vi "GetStatus.vi"(8 "error in (no error)":errorcluster, 11 "AODAcq in":refnum<class "AODAcq.lvclass">) -> (0 "error out":errorcluster, 2 "Status":T2, 3 "AODAcq out":refnum<class "AODAcq.lvclass">)   [LabVIEW 2011, in "AODAcq.lvclass"]
uses:
  AODAcq.lvclass
  FPGA_Control/FPGAState.ctl
  <vilib>/rvi/interface/RandomDataEmulation/niFpgaReadControlTemplate.vi
  <vilib>/rvi/interface/nirviReadWriteControl/nirviReadWriteControl.xnode
  FPGA_Control/AODRef.ctl
  FPGA_Control/AOD Control (FPGA).vi
panel:
  out "Status.TemporalChFull":bool
  out "Scan.NumPoints":u32
  out "Status.DownsampleDone":bool
  out "Status.MotionChFull":bool
  out "Status.ImChFull":bool
  out "Scan.NumMotionPoints":u32
  out "Scan.Motion Increment":u32
  out "Scan.TotalSamples":u32
  out "Debug.PMT_Unpacked_backlog":u32
  out "Debug.PMT_Data_backlog":u32
  out "AOD.UpdatesPerPoint":u32=2000
  out "Comm.CommLines":enum16{"1", "2", "4"}(ring)
  out "Comm.WriteCount":i32
  out "Comm.Written":cluster{"Address":u8, "Value":u32}[](array[cluster])
  out "Debug.Point":cluster{"X":i32, "Y":i32, "Z":i32}
  out "Status.BufferedPoints":i32
  out "Debug.PMT_Samples":u32
  out "Scan.Samples":u32
  out "Debug.PMT Array":i32[](array[numeric])
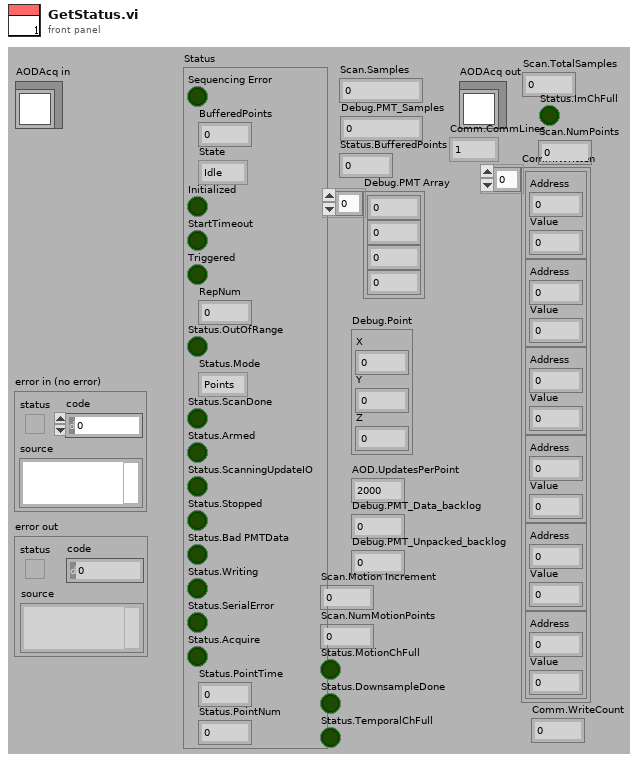
[diagram p1: front panel]
types:
  T1 = typedef "FPGAState.ctl" = enum16{"Idle", "Arm Scan", "Scan", "End Scan"}
  T2 = cluster{"Sequencing Error":bool, "BufferedPoints":i32, "State":T1, "Initialized":bool, "StartTimeout":bool, "Triggered":bool, "RepNum":u32, "Status.OutOfRange":bool, "Status.Mode":enum16{"Points", "Volume", "Idle"}, "Status.ScanDone":bool, "Status.Armed":bool, "Status.ScanningUpdateIO":bool, "Status.Stopped":bool, "Status.Bad PMTData":bool, "Status.Writing":bool, "Status.SerialError":bool, "Status.Acquire":bool, "Status.PointTime":u32, "Status.PointNum":u64}
  T3 = typedef "AODRef.ctl" = refnum<k20>
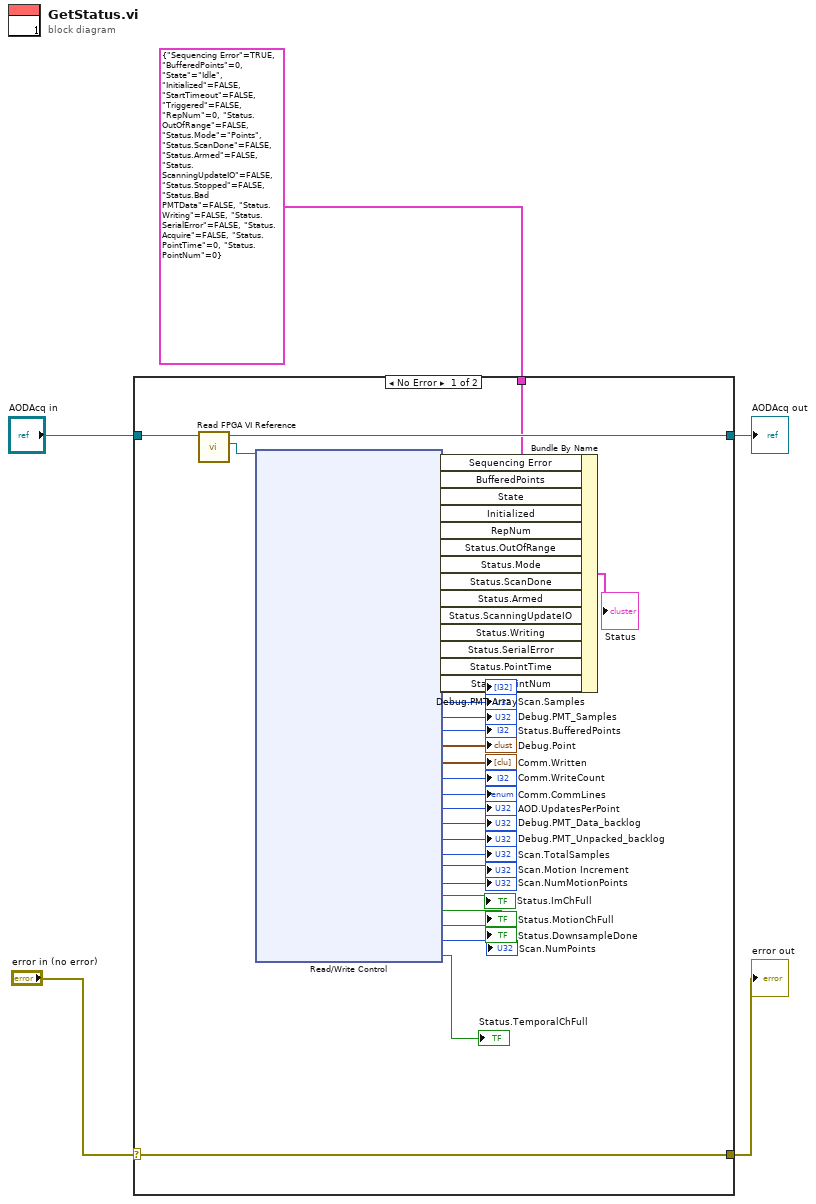
[diagram p0: block diagram]
diagram:
  n1 = case shown="No Error" "error in (no error)" {
    selector: "error in (no error)" -> [w44 w46]
    tunnel: [w44 w46] -> w4
    tunnel: [w42 w45] -> w2
    tunnel: "AODAcq in" -> [w43 w45]
    tunnel: T2 {"Sequencing Error"=TRUE, "BufferedPoints"=0, "State"=enum."Idle", "Initialized"=FALSE, "StartTimeout"=FALSE, "Triggered"=FALSE, "RepNum"=0, "Status.OutOfRange"=FALSE, "Status.Mode"=enum."Points", "Status.ScanDone"=FALSE, "Status.Armed"=FALSE, "Status.ScanningUpdateIO"=FALSE, "Status.Stopped"=FALSE, "Status.Bad PMTData"=FALSE, "Status.Writing"=FALSE, "Status.SerialError"=FALSE, "Status.Acquire"=FALSE, "Status.PointTime"=0, "Status.PointNum"=0} -> [w38 _]
    frame No Error {
      n2 = call-dynamic "Read FPGA VI Reference.vi"("AODAcq in"=w43) -> ("FPGA VI Reference"=w41:T3, "AODAcq out"=w42:refnum<class "AODAcq.lvclass">)  [unwired: 8 in, 1 out]
      n3 = xnode "Read/Write Control"("FPGA VI Reference In"=w41) -> ("Status.Sequencing error"=w40:bool, "Status.BufferedPoints"=w39:i32, "Status.State"=w37:T1, "Status.Initialized"=w36:bool, "Status.RepNum"=w35:u32, "Status.OutOfRange"=w34:bool, "Status.Mode"=w33:enum16{"Points", "Volume", "Idle"}, "Status.ScanDone"=w32:bool, "Status.Armed"=w31:bool, "Status.ScanUpdateIO"=w30:bool, "Status.Writing"=w27:bool, "Status.Serial error"=w6:bool, "Status.PointTime"=w28:u32, "Status.PointNum"=w29:u32, "Debug.PMT Array"=→"Debug.PMT Array":i32[], "Scan.Samples"=→"Scan.Samples":u32, "Debug.PMT_Samples"=→"Debug.PMT_Samples":u32, "Status.BufferedPoints"=→"Status.BufferedPoints":i32, "Debug.Point"=→"Debug.Point":cluster{"X":i32, "Y":i32, "Z":i32}, "Comm.Written"=→"Comm.Written":cluster{"Address":u8, "Value":u32}[], "Comm.WritenCount"=→"Comm.WriteCount":i32, "Comm.CommLines"=→"Comm.CommLines":enum16{"1", "2", "4"}, "AOD.UpdatesPerPoint"=→"AOD.UpdatesPerPoint":u32, "Debug.PMT_Data_backlog"=→"Debug.PMT_Data_backlog":u32, "Debug.PMT_Unpacked_backlog"=→"Debug.PMT_Unpacked_backlog":u32, "Scan.TotalSamples"=→"Scan.TotalSamples":u32, "Scan.Motion Increment"=→"Scan.Motion Increment":u32, "Scan.NumMotionPoints"=→"Scan.NumMotionPoints":u32, "Status.ImChFull"=→"Status.ImChFull":bool, "Status.MotionChFull"=→"Status.MotionChFull":bool, "Status.DownsampleDone"=→"Status.DownsampleDone":bool, "Scan.NumPoints"=→"Scan.NumPoints":u32, "Status.TemporalChFull"=→"Status.TemporalChFull":bool)  [unwired: 1 in, 2 out]
      n4 = Bundle By Name(cluster=w38, "Sequencing Error"=w40, "BufferedPoints"=w39, "State"=w37, "Initialized"=w36, "RepNum"=w35, "Status.OutOfRange"=w34, "Status.Mode"=w33, "Status.ScanDone"=w32, "Status.Armed"=w31, "Status.ScanningUpdateIO"=w30, "Status.Writing"=w27, "Status.SerialError"=w6, "Status.PointTime"=w28, "Status.PointNum"=w29) -> (→"Status":T2)
    }
    frame Error {
    }
  }
  "error out" <- w4
  "AODAcq out" <- w2
